vi "LINEAR.vi"(1 "I":dbl, 2 "N":dbl, 3 "END":dbl, 4 "INITIAL":dbl) -> (0 "数值":dbl)   [LabVIEW 2017]
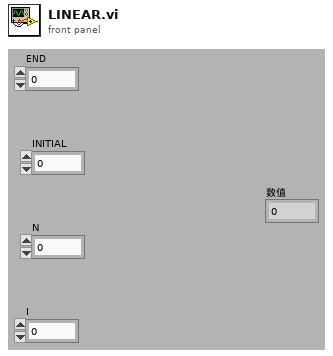
[diagram p1: front panel]
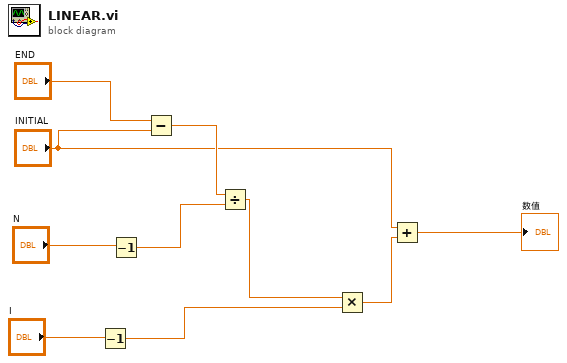
[diagram p0: block diagram]
diagram:
  n1 = Decrement(x="I") -> (x-1=w5:dbl)
  n2 = Decrement(x="N") -> (x-1=w7:dbl)
  n3 = Subtract(x="END", y="INITIAL") -> (x-y=w8:dbl)
  n4 = Divide(x=w8, y=w7) -> (x/y=w4:dbl)
  n5 = Multiply(x=w4, y=w5) -> (x*y=w2:dbl)
  n6 = Add(x="INITIAL", y=w2) -> (x+y=→"数值":dbl)
